vi "SetAcquisitions.vi"(8 "error in":errorcluster, 10 "Acquisitions":u64, 11 "camera in":refnum<class "camera.lvclass">) -> (0 "error out":errorcluster)   [LabVIEW 2020, in "camera.lvclass"]
uses:
  camera.lvclass
  camera.lvclass/camera.ctl
  lib/O-PL.dll
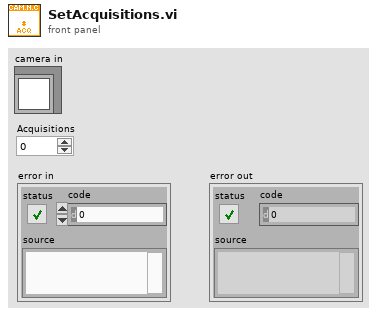
[diagram p1: front panel]
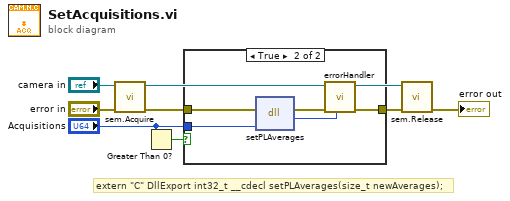
[diagram p0: block diagram]
diagram:
  # "extern \"C\" DllExport int32_t __cdecl setPLAverages(size_t newAverages);"
  n1 = call "sem.Acquire.vi"("error in"="error in", "camera.nit in"="camera in") -> ("error out"=w7:errorcluster)  [unwired: 9 in]
  n2 = Greater Than 0?(x="Acquisitions") -> (x > 0?=w5:bool)
  n3 = case shown="True" w5 {
    tunnel: "Acquisitions" -> [_ w12]
    tunnel: w7 -> [w8 w13]
    tunnel: [w8 w9] -> w6
    frame False {
    }
    frame True {
      n4 = dll-call lib="C:/Users/pittsburger.SOLARIS/Desktop/v0.8/lib/O-PL.dll" fn="setPLAverages"(error in=w13, "newAverages"=w12) -> (error out=w11:errorcluster, "return"=w10:i32)  [unwired: 3 in, 1 out]
      n5 = call "errorHandler.vi"("code"=w10, "error in"=w11) -> ("error out"=w9:errorcluster)  [unwired: 9 in]
    }
  }
  n6 = call "sem.Release.vi"("error in"=w6, "camera.nit in"="camera in") -> ("error out"=→"error out":errorcluster)  [unwired: 9 in]
